vi "GetArray.vi"(4 "Sequence Context":T1) -> (0 "error out":errorcluster, 1 "Test Data":T2 {"Numeric Measurement" format="%.2f"})   [LabVIEW 2010]
uses:
  <vilib>/addons/TestStand/_TSLegacy.llb/LabVIEW Test - Test Data.ctl
  <vilib>/addons/TestStand/_TSLegacy.llb/LabVIEW Test - Sequence Context.ctl
  <vilib>/Analysis/NI_AALBase.lvlib
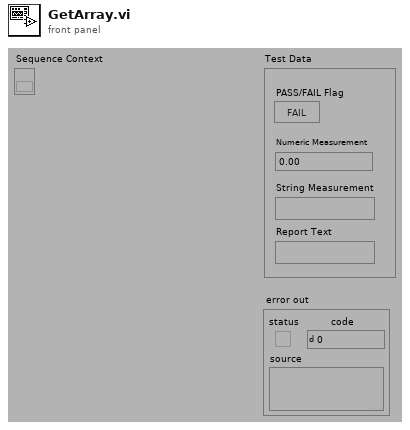
[diagram p1: front panel]
types:
  T1 = typedef "LabVIEW Test - Sequence Context.ctl" = refnum<k7>
  T2 = typedef "LabVIEW Test - Test Data.ctl" = cluster{"PASS/FAIL Flag":bool, "Numeric Measurement":dbl, "String Measurement":string, "Report Text":string}
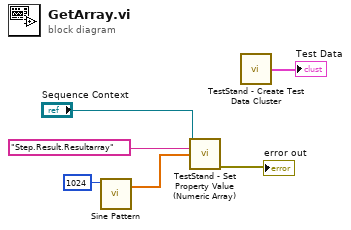
[diagram p0: block diagram]
diagram:
  n1 = call <vilib>:"Sine Pattern.vi"("samples"=1024) -> ("Sinusoidal Pattern"=w2:dbl[])  [unwired: 3 in, 1 out]
  n2 = call <vilib>:"TestStand - Set Property Value (Numeric Array).vi"("Sequence Context In"="Sequence Context", "Lookup String"="Step.Result.Resultarray", "New Value"=w2) -> ("error out"=→"error out":errorcluster)  [unwired: 2 in, 10 out]
  n3 = call "TestStand - Create Test Data Cluster.vi"() -> ("Test Data"=→"Test Data":T2)  [unwired: 4 in]
